vi "close.vi"(11 "Experience ID":string) -> (0 "error out":errorcluster)   [LabVIEW 2015]
panel:
  # "Close"
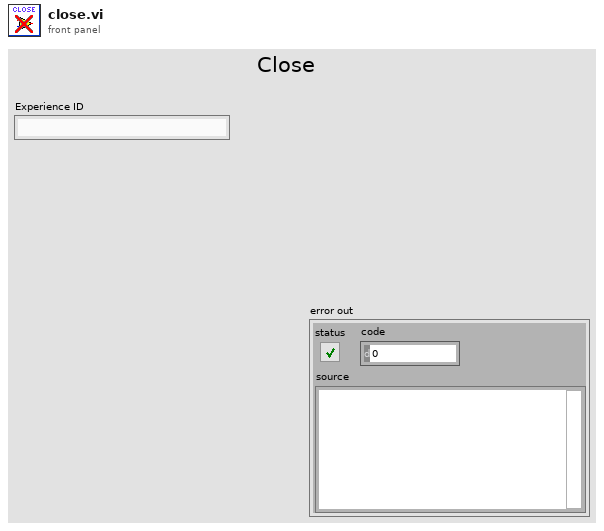
[diagram p1: front panel]
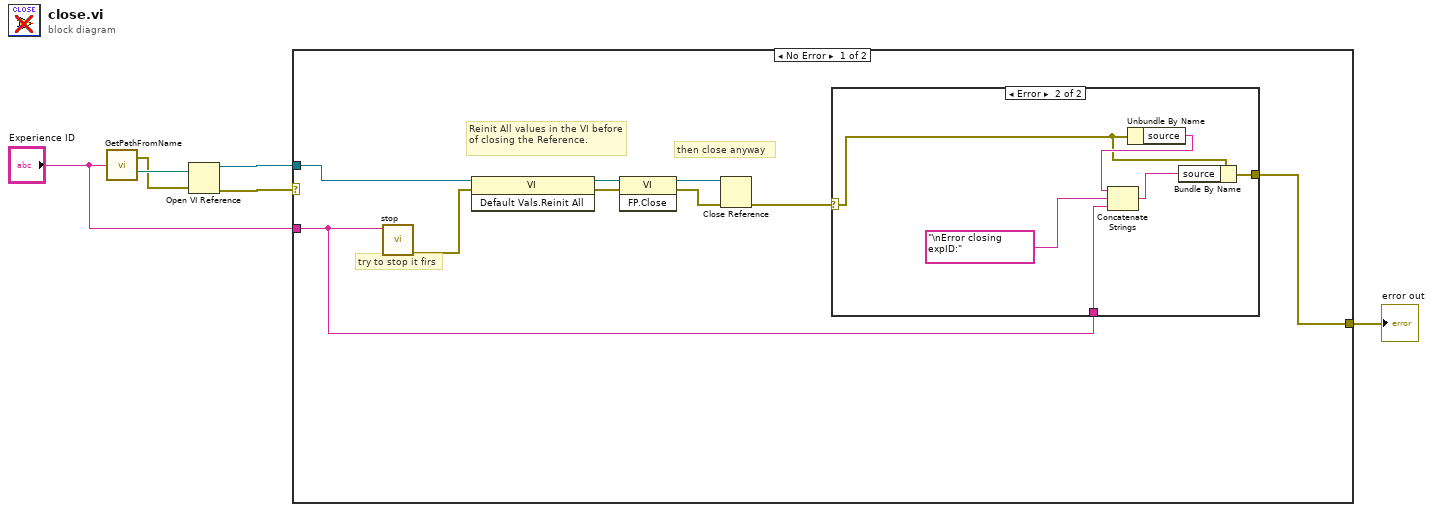
[diagram p0: block diagram]
diagram:
  n1 = call "GetPathFromName.vi"("Experience ID"="Experience ID") -> ("Error out"=w5:errorcluster, "VI_Path"=w6:path)
  n2 = Open VI Reference(vi path=w6, error in (no error)=w5) -> (vi reference=w2:refnum<vi>, error out=w3:errorcluster)  [unwired: 1 in, 3 out]
  n3 = case shown="No Error" w3 {
    selector: w3 -> [_ w23]
    tunnel: [w7 w23] -> w4
    tunnel: w2 -> [w10 _]
    tunnel: "Experience ID" -> [w8 _]
    frame No Error {
      # "try to stop it firs"
      # "then close anyway"
      # "Reinit All values in the VI before of closing the Reference."
      n4 = call "stop.vi"("Experience ID"=w8) -> ("error out"=w11:errorcluster)  [unwired: 10 in]
      n5 = invoke class="VI" method="Default Vals.Reinit All"(reference=w10, error in=w11) -> (reference out=w15:refnum<vi>, error out=w14:errorcluster)  [unwired: 1 in, 1 out]
      n6 = invoke class="VI" method="FP.Close"(reference=w15, error in=w14) -> (reference out=w13:refnum<vi>, error out=w12:errorcluster)  [unwired: 1 in, 1 out]
      n7 = Close Reference(reference=w13, error in (no error)=w12) -> (error out=w9:errorcluster)
      n8 = case shown="Error" w9 {
        selector: w9 -> [w16 w18]
        tunnel: [w16 w22] -> w7
        tunnel: w8 -> [_ w17]
        frame No Error {
        }
        frame Error {
          n9 = Unbundle By Name(w18) -> ("source"=w21:string)
          n10 = Concatenate Strings(w21, "\nError closing expID:" ("FailDescriptor"), w17) -> (w20:string)
          n11 = Bundle By Name(cluster=w18, "source"=w20) -> (w22:errorcluster)
        }
      }
    }
    frame Error {
    }
  }
  "error out" <- w4
